vi "FTW-Actor-CheckShutdown.vi"(0 "FTW Actor Instance":refnum<class "FTW-Actor-Instance.lvclass">, 11 "error in":errorcluster) -> (4 "FTW Actor Instance out":refnum<class "FTW-Actor-Instance.lvclass">, 8 "Shutdown?":bool, 15 "error out":errorcluster)   [LabVIEW 2015, in "FTW-Actor-Instance.lvclass"]
uses:
  FTW-Actor-Instance.lvclass
  FTW-Actor-Instance.lvclass/FTW-Actor-Instance.ctl
  scheduler/FTW-Scheduler.lvclass
panel:
  # "Inputs"
  # "Outputs"
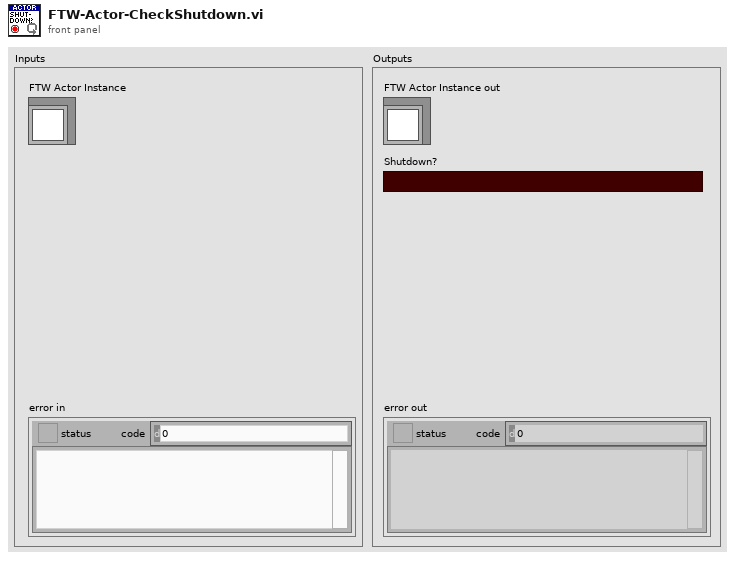
[diagram p1: front panel]
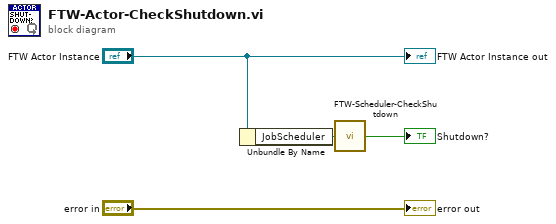
[diagram p0: block diagram]
diagram:
  n1 = Unbundle By Name("FTW Actor Instance") -> ("JobScheduler"=w3:refnum<class "FTW-Scheduler.lvclass">)
  n2 = call "FTW-Scheduler-CheckShutdown.vi"("FTW Job Scheduler"=w3) -> ("Shutdown?"=→"Shutdown?":bool)
  "error out" <- "error in"
  "FTW Actor Instance out" <- "FTW Actor Instance"
